vi "End Run.vi"(8 "abort":bool, 11 "NetCPU in":refnum<class "NetCPU.lvclass">) -> (3 "NetCPU out":refnum<class "NetCPU.lvclass">)   [LabVIEW 2020, in "NI_TargetHelper.lvlib" / "NetCPU.lvclass"]
uses:
  <vilib>/TargetSupport/NI_TargetHelper/NetCPU/NetCPU.lvclass
  <vilib>/TargetSupport/NI_TargetHelper/NetCPU/NetCPU.lvclass/NetCPU.ctl
  <vilib>/TargetSupport/NI_TargetHelper/Run Target VI.ctl
  <vilib>/TargetSupport/NI_TargetHelper/Instance VIref.ctl
  <vilib>/TargetSupport/NI_TargetHelper/NI_TargetHelper.lvlib
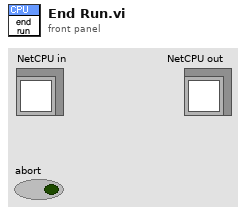
[diagram p1: front panel]
types:
  T1 = typedef "NI_TargetHelper.lvlib/Instance VIref.ctl" = refnum<vi>
  T2 = typedef "NI_TargetHelper.lvlib/Run Target VI.ctl" = refnum<vi>
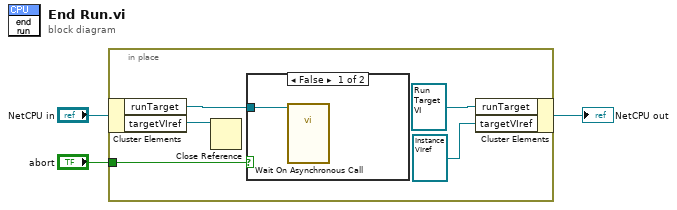
[diagram p0: block diagram]
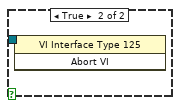
[diagram p2: hidden frame]
diagram:
  n1 = in-place {
    in-place-border: "abort" -> [w7]
    n2 = in-place-cluster #1("NetCPU in") -> ("runTarget"=w8:T2, "targetVIref"=w4:T1)
    n3 = Close Reference(reference=w4) -> ()  [unwired: 1 in, 1 out]
    n4 = case shown="False" w7 {
      tunnel: w8 -> [w9 w10]
      frame False {
        n5 = call-by-ref "Wait On Asynchronous Call"(reference=w9) -> ()  [unwired: 13 in, 2 out]
      }
      frame True {
        n6 = invoke class="VI Interface Type 125" method="Abort VI"(reference=w10) -> ()  [unwired: 2 in, 3 out]
      }
    }
    n7 = in-place-cluster #1("runTarget"=T2 refnum, "targetVIref"=T1 refnum) -> (→"NetCPU out":refnum<class "NetCPU.lvclass">)
  }
